vi "FruitCaught.vi"(0 "object in":refnum<class "Game Board.lvclass">, 5 "error in (no error)":errorcluster) -> (14 "object out":refnum<class "Game Board.lvclass">, 15 "Fruit Caught?":bool, 19 "error out":errorcluster)   [LabVIEW 2021, in "Game Board.lvclass"]
uses:
  Game Board.lvclass
  Game Board.lvclass/Game Board.ctl
  Snake_class/Snake.lvclass
  Fruit_class/Fruit.lvclass
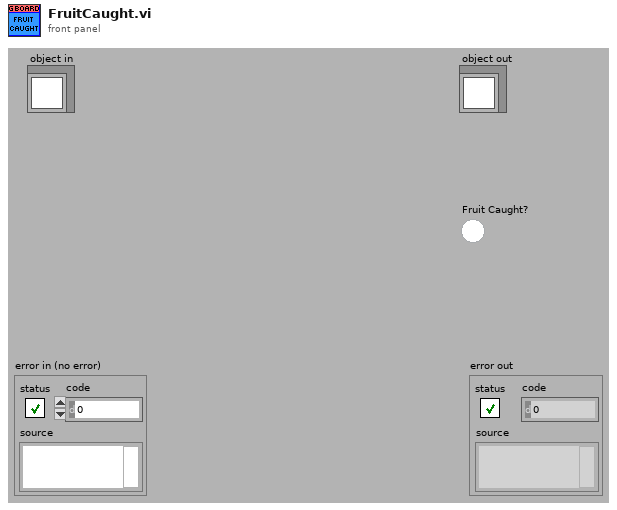
[diagram p1: front panel]
types:
  T1 = typedef "Coordinates.ctl" = cluster{"X":i32, "Y":i32}
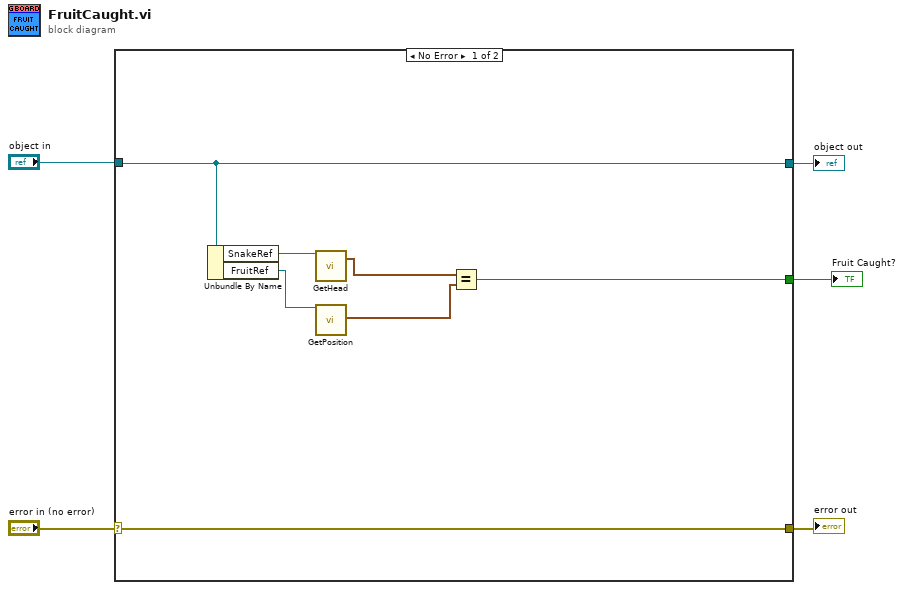
[diagram p0: block diagram]
diagram:
  n1 = case shown="No Error" "error in (no error)" {
    selector: "error in (no error)" -> [w12 w14]
    tunnel: [w12 w14] -> w4
    tunnel: [w11 w13] -> w2
    tunnel: "object in" -> [w11 w13]
    tunnel: [w6 _] -> w1
    frame No Error {
      n2 = Unbundle By Name(w11) -> ("SnakeRef"=w10:refnum<class "Snake.lvclass">, "FruitRef"=w9:refnum<class "Fruit.lvclass">)
      n3 = call-dynamic "GetHead.vi"("object in"=w10) -> ("Head"=w8:T1)  [unwired: 16 in, 2 out]
      n4 = call "GetPosition.vi"("object in"=w9) -> ("Coordinates"=w7:T1)  [unwired: 17 in, 1 out]
      n5 = Equal?(x=w8, y=w7) -> (x = y?=w6:bool)
    }
    frame Error {
    }
  }
  "error out" <- w4
  "object out" <- w2
  "Fruit Caught?" <- w1
